vi "Read Buffer Size.vi"(11 "Template in":refnum<class "Template.lvclass">) -> (3 "EDVR Pool Size":i32)   [LabVIEW 2020, in "Template.lvlib" / "Template.lvclass"]
uses:
  Template.lvclass
  Template.lvclass/Template.ctl
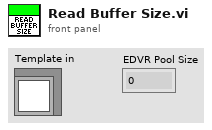
[diagram p1: front panel]
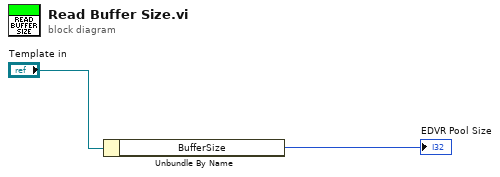
[diagram p0: block diagram]
diagram:
  n1 = Unbundle By Name("Template in") -> ("BufferSize"=→"EDVR Pool Size":i32)
